vi "GCS3_Prepare_Motion_Error.vi"(0 "System no.":i32=1 min=1 max=4 step=1, 2 "Axis (ContainerUnit)":string, 3 "PID controller (FunctionUnit)":string, 5 "error in":errorcluster) -> (14 "Axis Parameter Configuration":T1[](array[typedef]), 16 "Original PID values":string[](array[string]), 19 "error out":errorcluster)   [LabVIEW 2026]
doc: "Prepares a PI GCS 3.0 system for motion error by setting the PID parameters to zero. This is only a sample. Do not use in production code.\n\nCompatibility: This sample requires a PI GCS 3.0 controller."
uses:
  SpecialCommand/UserCommandLevel.ctl
  GeneralCommands/ParameterInfoSet.ctl
panel:
  # "Prepares a PI GCS 3.0 system for motion error by setting the PID parameters to zero.\nThis is only a sample. Do not use in production code.\n\nCompatibility: This sample requires a PI GCS 3.0 controller."
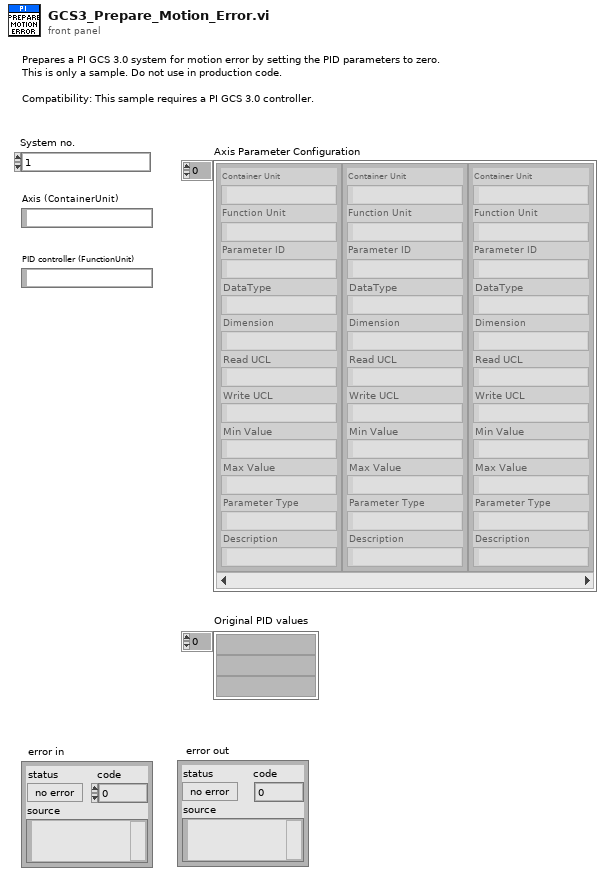
[diagram p1: front panel]
types:
  T1 = typedef "ParameterInfoSet.ctl" = cluster{"Container Unit":string, "Function Unit":string, "Parameter ID":string, "DataType":string, "Dimension":string, "Read UCL":string, "Write UCL":string, "Min Value":string, "Max Value":string, "Parameter Type":string, "Description":string}
  T2 = typedef "UserCommandLevel.ctl" = enum16{"User", "Expert", "PI Staff", "FW Developer"}
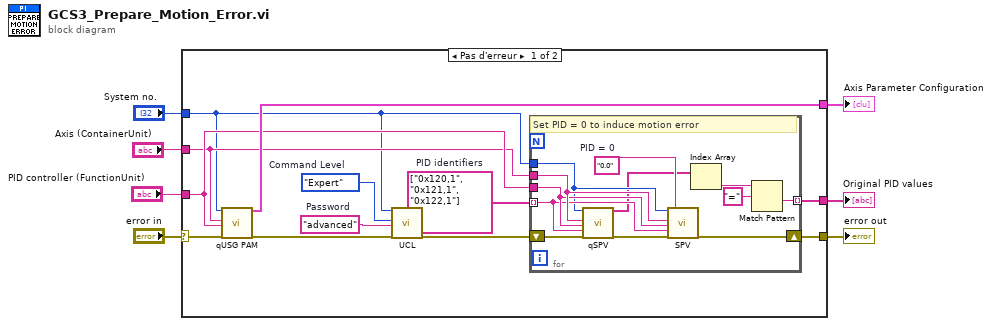
[diagram p0: block diagram]
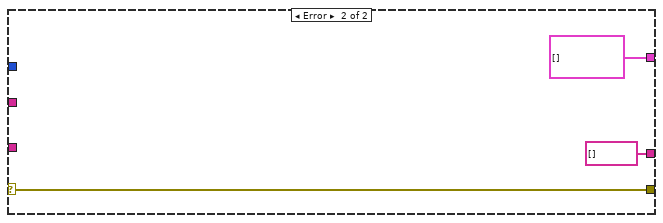
[diagram p2: hidden frame]
diagram:
  n1 = case shown="Pas d'erreur" "error in" {
    selector: "error in" -> [w11 w34]
    tunnel: [w19 T1[] [] ("Array of ParametersInfo")] -> w7
    tunnel: "PID controller (FunctionUnit)" -> [w15 _]
    tunnel: [w14 string[] []] -> w1
    tunnel: "Axis (ContainerUnit)" -> [w13 _]
    tunnel: [w12 w34] -> w6
    tunnel: "System no." -> [w8 _]
    frame No Error {
      w9 = UserCommandLevel."Expert"  # Command Level
      w10 = string[] ["0x120,1", "0x121,1", "0x122,1"]  # PID identifiers
      w18 = "advanced"  # Password
      n2 = call "qUSG PAM.vi"("System no."=w8, "ContainerUnit"=w13, "FunctionUnit"=w15, "error in"=w11) -> ("Array of ParametersInfo"=w19:T1[], "error out"=w17:errorcluster)  [unwired: 14 in]
      n3 = call "UCL.vi"("System no."=w8, "Command Level"=w9, "Password"=w18, "error in"=w17) -> ("error out"=w16:errorcluster)  [unwired: 15 in]
      n4 = for {
        tunnel: w10 -> [w26] mode=indexing
        shift-right: [w29] -> w12
        shift-left: w16 -> [w31]
        tunnel: w13 -> [w28]
        tunnel: w15 -> [w27]
        tunnel: [w20] -> w14 mode=indexing
        tunnel: w8 -> [w24]
        w25 = "0.0"  # PID = 0
        # "Set PID = 0 to induce motion error"
        n5 = call "qSPV.vi"("System no."=w24, "ContainerUnit"=w28, "FunctionUnit"=w27, "ParameterID"=w26, "error in"=w31) -> ("Values"=w21:string[], "error out"=w30:errorcluster)  [unwired: 13 in]
        n6 = call "SPV.vi"("System no."=w24, "ParameterSet"=w28, 3:w27, 4:w26, "error in"=w30, 6:w25) -> ("error out"=w29:errorcluster)  [unwired: 13 in]
        n7 = Index Array(array=w21) -> (element=w23:string)  [unwired: 1 in]
        n8 = Match Pattern(string=w23, regular expression="=") -> (after substring=w20:string)  [unwired: 1 in, 3 out]
      }
    }
    frame Error {
    }
  }
  "error out" <- w6
  "Axis Parameter Configuration" <- w7
  "Original PID values" <- w1
